vi "HLR_Scale and Mean 1d.vi"(10 "Slope & Offset":dbl[][](array[numeric]), 11 "Raw In":dbl[](array[numeric])) -> (2 "Scaled Value":dbl[](array[numeric]))   [LabVIEW 2025]
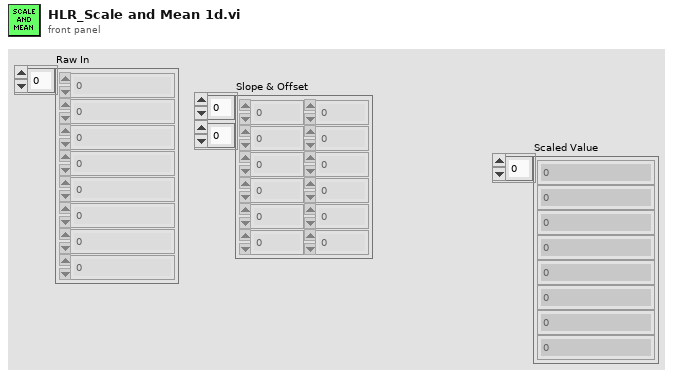
[diagram p1: front panel]
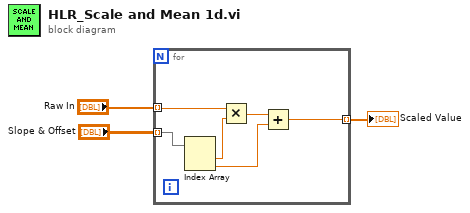
[diagram p0: block diagram]
diagram:
  n1 = for {
    tunnel: "Raw In" -> [w9] mode=indexing
    tunnel: [w4] -> w3 mode=indexing
    tunnel: "Slope & Offset" -> [w8] mode=indexing
    n2 = Index Array(array=w8) -> (element #1=w7:dbl, element #2=w5:dbl)  [unwired: 2 in]
    n3 = Multiply(x=w9, y=w7) -> (x*y=w6:dbl)
    n4 = Add(x=w6, y=w5) -> (x+y=w4:dbl)
  }
  "Scaled Value" <- w3
